vi "Ethernet-II-Create.vi"(6 "Add CRC32?":bool, 7 "PadLen?":bool=TRUE, 8 "Payload (in)":u8[](array[numeric])=[0, 1, 8, 0, 6, 4, 0, 1, 0, 35, 38, 182, 175, 53, 192, 168, 1, 200, 0, 0, 0, 0, 0, 0, 192, 168, 1, 201, 0, 0, 0, 0, 0, 0, 0, 0, 0, 0, 0, 0, 0, 0, 0, 0, 0, 0] format="%02x", 9 "EtherType":u16=2054 format="%04x", 10 "Source MAC":u8[](array[numeric])=[0, 35, 38, 182, 175, 53] format="%02x", 11 "Destination MAC":u8[](array[numeric])=[255, 255, 255, 255, 255, 255] format="%02x") -> (3 "Ethernet Frame (out)":u8[](array[numeric]) format="%02x")   [LabVIEW 2018]
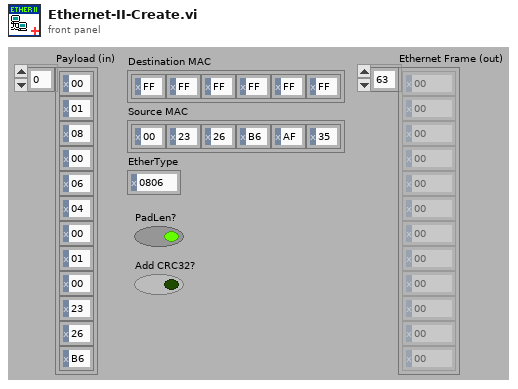
[diagram p1: front panel]
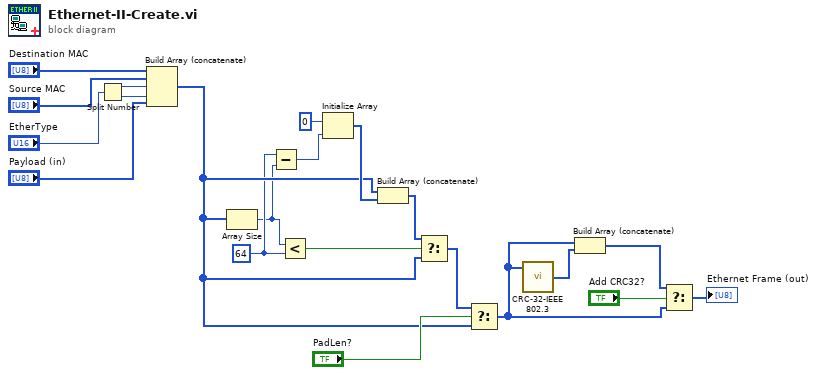
[diagram p0: block diagram]
diagram:
  w7 = 64 ("y")
  n1 = Split Number(x="EtherType") -> (hi(x)=w18:u8, lo(x)=w17:u8)
  n2 = Build Array (concatenate)("Destination MAC", "Source MAC", w18, w17, "Payload (in)") -> (w8:u8[])
  n3 = Array Size(array=w8) -> (size(s)=w6:i32)
  n4 = Subtract(x=w7, y=w6) -> (x-y=w11:i32)
  n5 = Less?(x=w6, y=w7) -> (x < y?=w15:bool)
  n6 = Initialize Array(u8 0, w11) -> (w13:u8[])
  n7 = Build Array (concatenate)(w8, w13) -> (w14:u8[])
  n8 = Select(t=w14, s=w15, f=w8) -> (s? t:f=w10:u8[])
  n9 = Select(t=w10, s="PadLen?", f=w8) -> (s? t:f=w1:u8[])
  n10 = call "CRC-32-IEEE 802.3.vi"("Frame in"=w1) -> ("CRC32[]"=w5:u8[])  [unwired: 3 in, 1 out]
  n11 = Build Array (concatenate)(w1, w5) -> (w3:u8[])
  n12 = Select(t=w3, s="Add CRC32?", f=w1) -> (s? t:f=→"Ethernet Frame (out)":u8[])
